vi "002_WarningLog.vi"(11 "Queue Ref":T1={"UI"=refnum, "Message"=refnum, "Data"=refnum, "Caller"=refnum, "Name"="000 Common", "Data Path"=path "", "Class Path"=path "", "SubPanel"=refnum, "Project Name"="", "MNT"="", "Title"="", "Data Source"=refnum, "Queue List"={}, "VI"=refnum, "UE"=refnum}) -> ()   [LabVIEW 2020]
uses:
  Alin/QMH/000 Module Data Type.ctl
  Alin/QMH/Queue Message.ctl
  9999 SubVI/Global/Data Global/Data Global Mode.ctl
  <vilib>/Utility/miscctls.llb/LVRowAndColumnUnsignedTypeDef.ctl
  9999 SubVI/Global/Data Global/SDQ Data Type.ctl
  <vilib>/Utility/file.llb/Read Delimited Spreadsheet (string).vi
panel:
  out "QN":i32
  out "Log Title":bool
  out "Warning Title":bool
  in  "Log Select":enum32{"History", "Real"}(radio)
  in  "Search Log":bool
  in  "Log Stop Time":timestamp caption="结束时间" format="%<%x %.0X>T"
  in  "Log Start Time":timestamp caption="开始时间" format="%<%x %.0X>T"
  in  "Warning Edit":bool
  in  "Warning Query":bool
  in  "Warning Stop Time":timestamp caption="结束时间" format="%<%x %X>T"
  in  "Warning Start Time":timestamp caption="开始时间" format="%<%x %.0X>T"
  in  "Warning Select":enum32{"History", "Real"}(radio)
  in  "Panel Show":bool
  in  "Operate":i32(listbox) caption="操作日志"
  in  "Warning":i32(listbox) caption="报警日志"
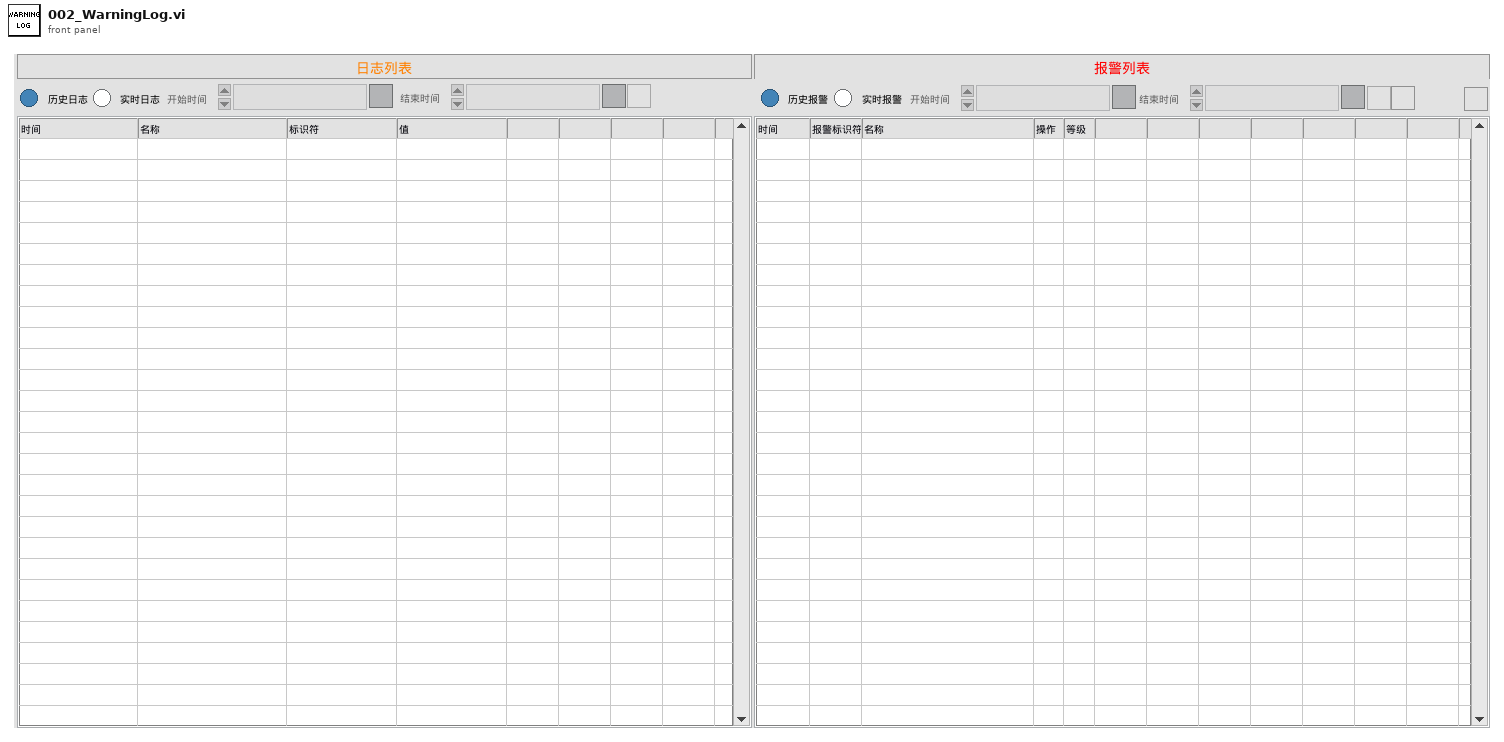
[diagram p1: front panel]
types:
  T1 = typedef "000 Module Data Type.ctl" = cluster{"UI":refnum<queue>, "Message":refnum<queue>, "Data":refnum<queue>, "Caller":refnum<queue>, "Name":string, "Data Path":path, "Class Path":path, "SubPanel":refnum<vi>, "Project Name":string, "MNT":string, "Title":string, "Data Source":refnum<queue>, "Queue List":map{string, refnum<queue>}, "VI":refnum<vi>, "UE":refnum<user-event>}
  T2 = typedef "SDQ Data Type.ctl" = cluster{"CAN Length":string, "CAN Name":string, "CAN ID":string, "CAN Type":string, "Test Item":string, "Byte Order":string, "Instruction":string, "Control Type":string, "Group":string, "Offset":dbl, "Coefficient":dbl, "Write Enable":bool, "Lable Type":string, "Key?":string, "Set Value":string, "Upper":dbl, "Lower":dbl, "Unit":string, "Formula":string, "Test Item Type":string, "Length":i32, "Address":string, "Name":string, "Identifier":string, "Data Type":string, "Enumerate?":string, "Enumerate List":string, "Data":string, "Source":string}
  T3 = cluster{"Queue Ref":T1, "Receive Data":map{string, T2}, "Log":string[][], "History Log":string[][], "Warning":string[][], "History Warning":string[][], "Delay":cluster{"Count Time(ms)":u32, "Delay Time(ms)":u32}, "Step":cluster{"Warning Judge":string, "Delay":string}}
  T4 = typedef "LVRowAndColumnUnsignedTypeDef.ctl" = cluster{"Row":u32, "Column":u32}
  T5 = enum8{"Enabled", "Disabled", "Disabled and Grayed Out"}
  T6 = typedef "eventvkey.ctl" = enum16{"ASCII", "Enter", "Return", "Shift", "Ctrl", "Alt", "Cmd", "Opt", "Caps", "NumLock", "Clear", "Break", "Up", "Down", "Left", "Right", "Insert", "Delete", "Home", "End", "PageUp", "PageDown", "Escape", "Help", "Pause", "ScrollLock", "F1", "F2", "F3", "F4", "F5", "F6", "F7", "F8", "F9", "F10", "F11", "F12", "F13", "F14", "F15", "F16", "F17", "F18", "F19", "F20", "F21", "F22", "F23", "F24", "Play", "VolumeUp", "VolumeDown", "Mute", "Two Byte Char"}
  T7 = cluster{"Shift":bool, "Ctrl":bool, "Alt":bool, "Cmd":bool, "Opt":bool}
  T8 = cluster{"Queue List":map{string, refnum<queue>}, "SubPanel":refnum<vi>, "Active Panel":string, "Queue Ref":T1, "Project Name":string}
  T9 = typedef "Data Global Mode.ctl" = enum16{"Init", "Read", "Write", "Write Data", "Load"}
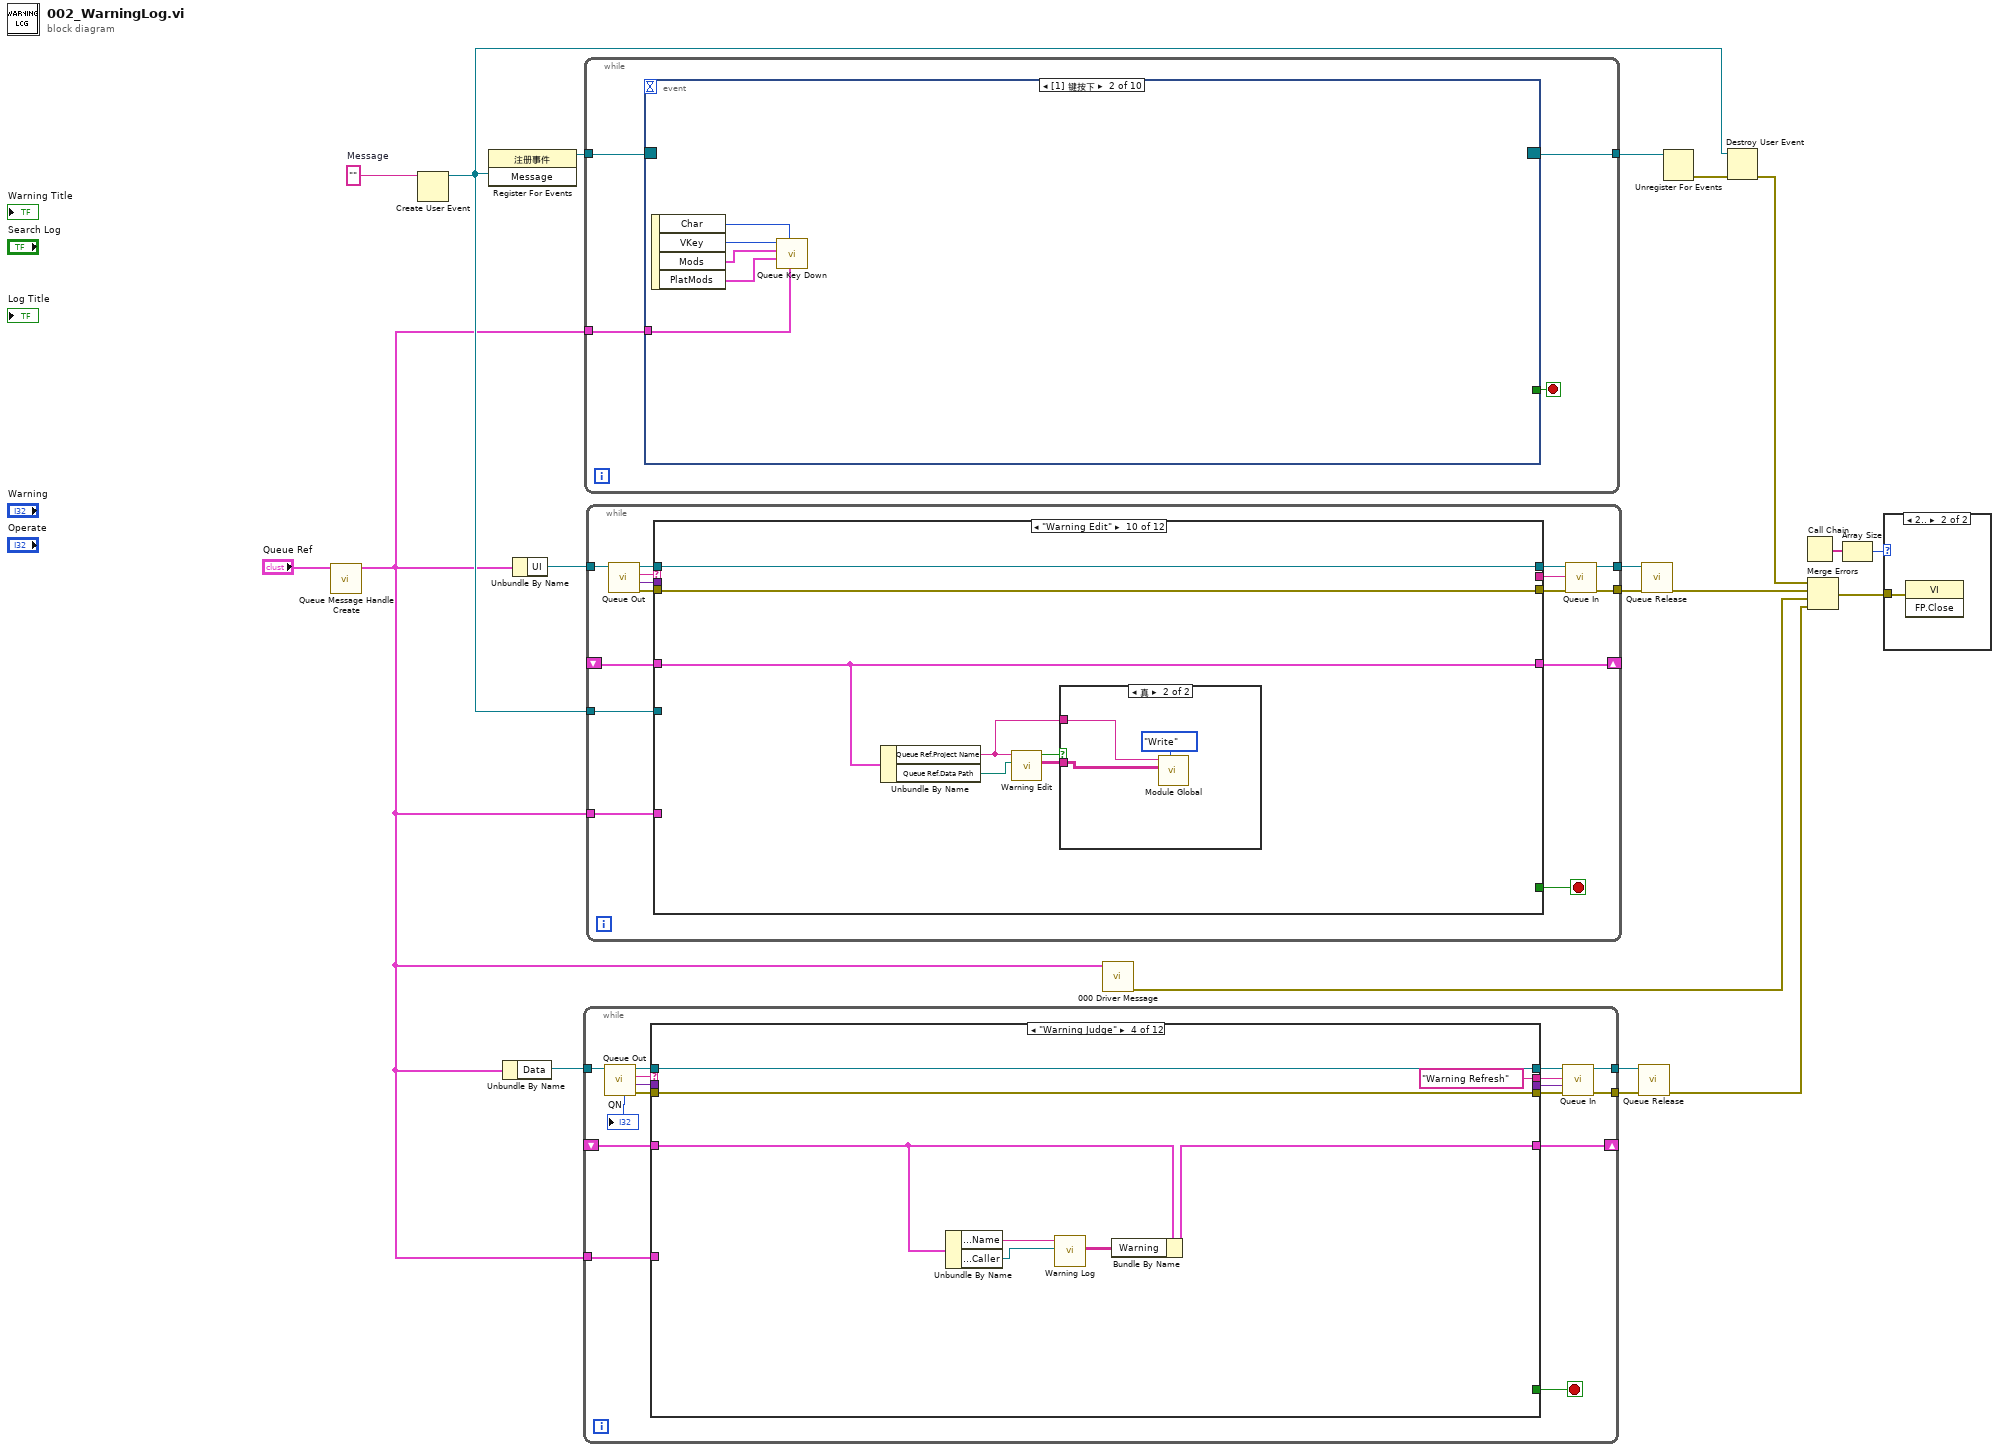
[diagram p0: block diagram]
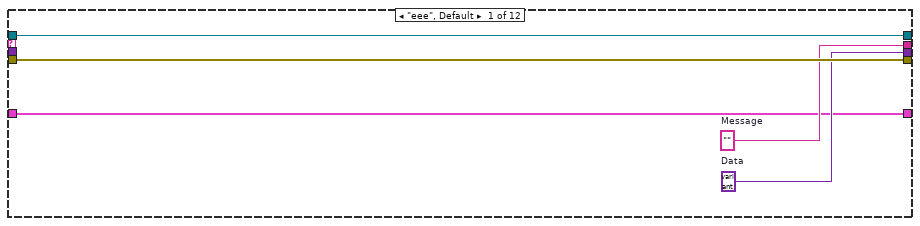
[diagram p2: hidden frame]
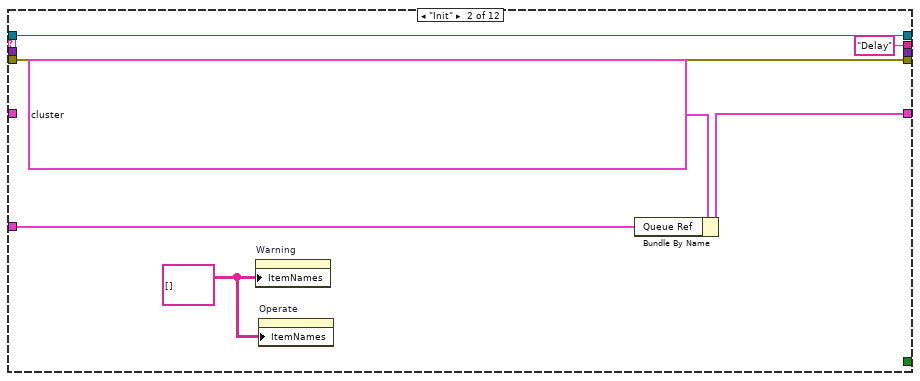
[diagram p3: hidden frame]
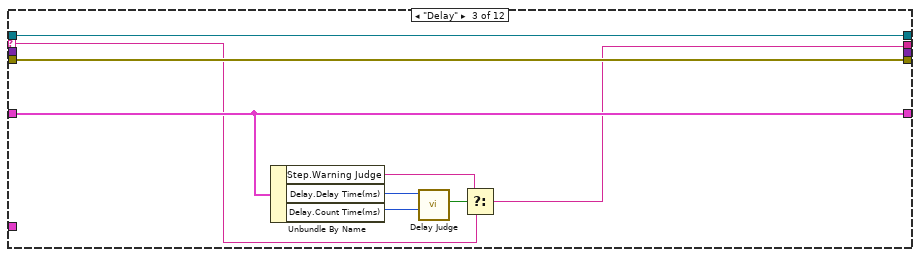
[diagram p4: hidden frame]
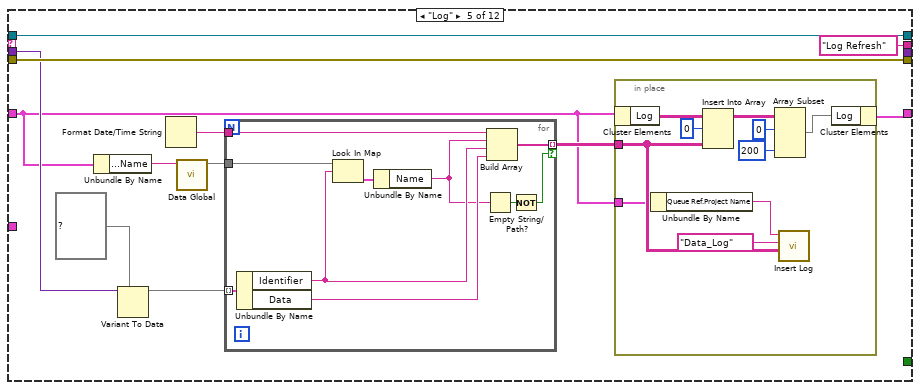
[diagram p5: hidden frame]
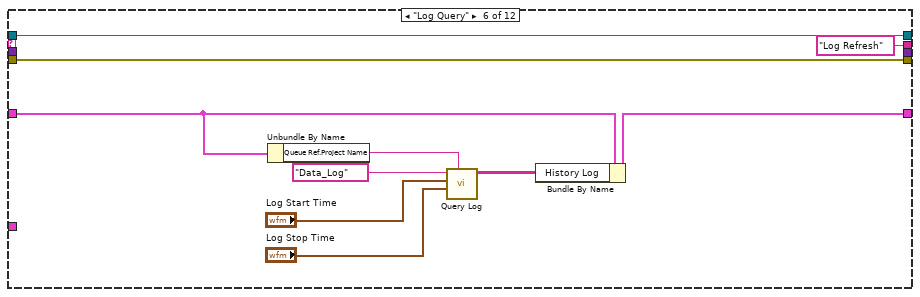
[diagram p6: hidden frame]
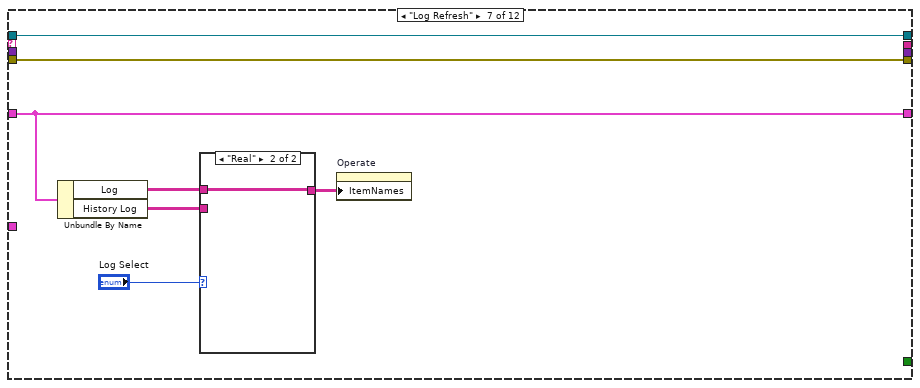
[diagram p7: hidden frame]
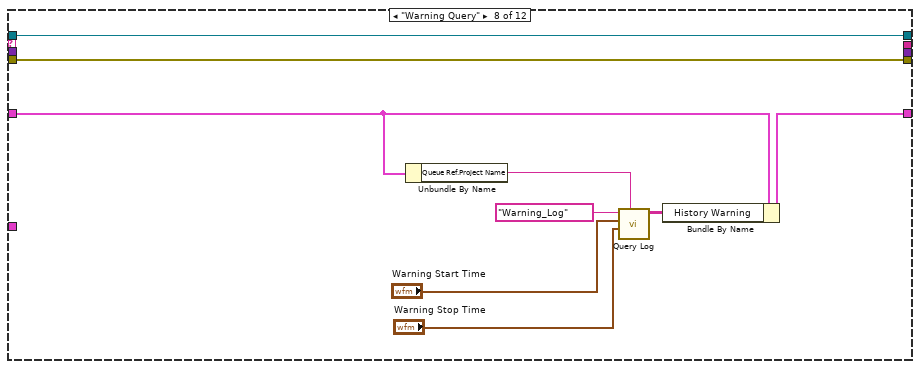
[diagram p9: hidden frame]
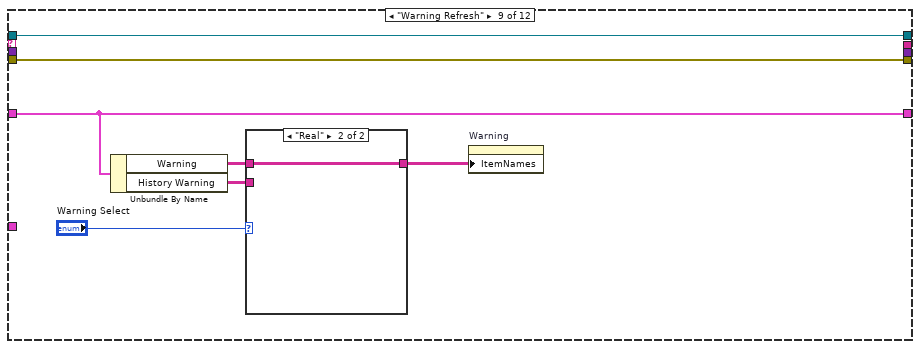
[diagram p10: hidden frame]
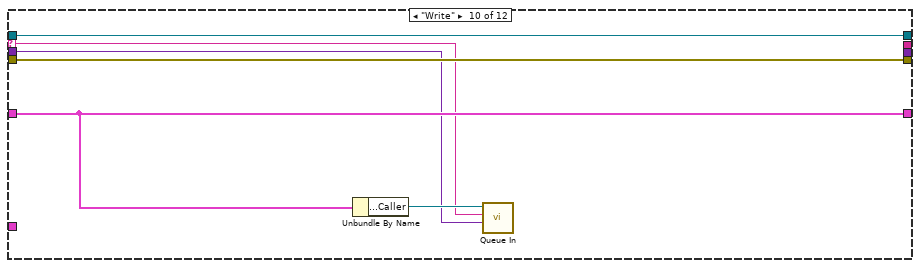
[diagram p12: hidden frame]
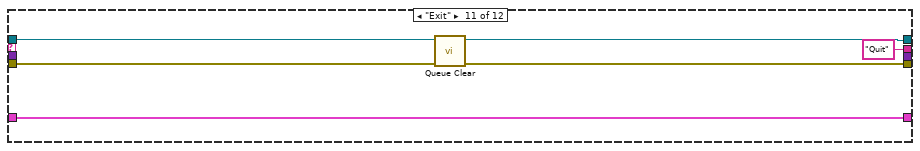
[diagram p13: hidden frame]
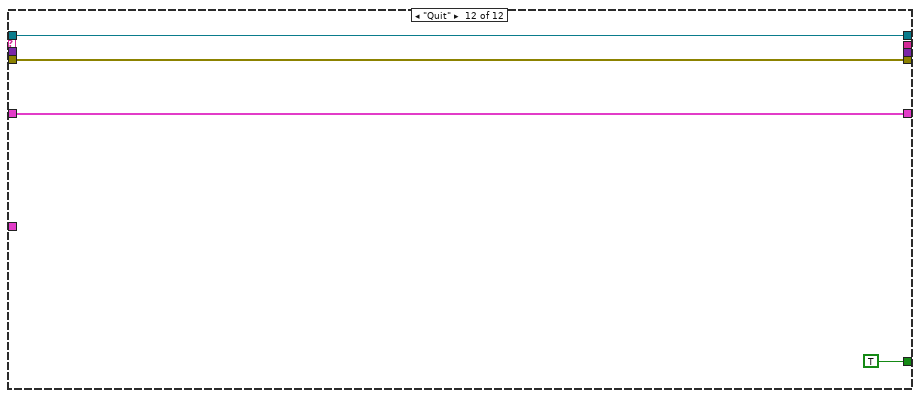
[diagram p14: hidden frame]
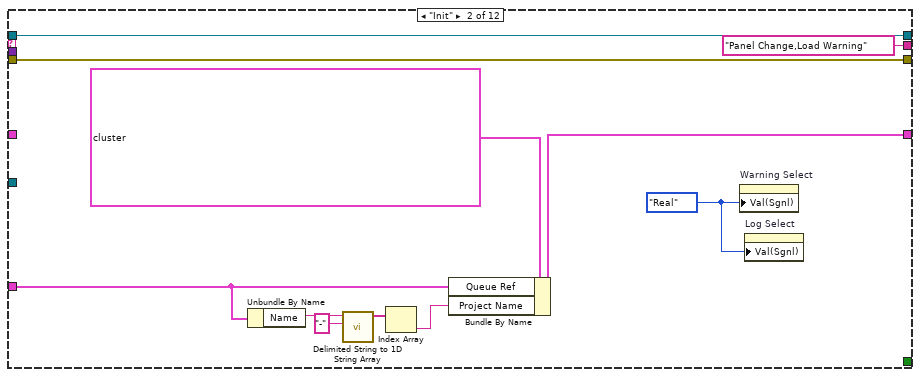
[diagram p17: hidden frame]
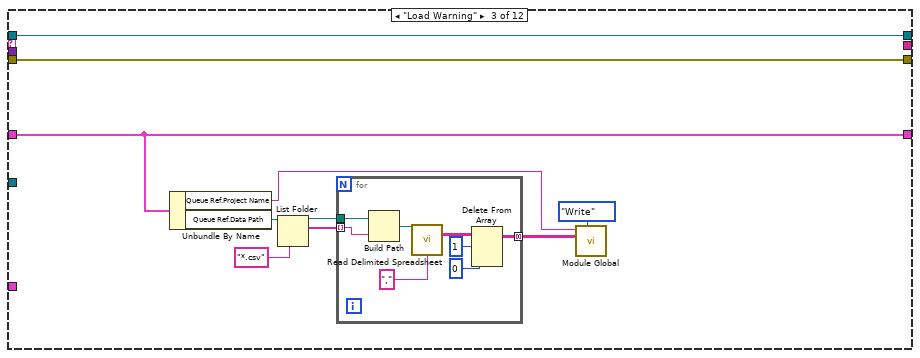
[diagram p18: hidden frame]
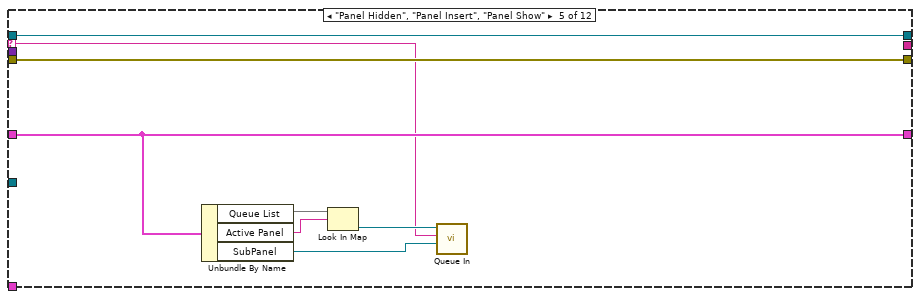
[diagram p20: hidden frame]
diagram:
  w3 = ""  # Message
  n1 = call "Queue Message Handle Create.vi"("Queue Ref In"="Queue Ref") -> ("Queue Ref Out"=w2:T1)  [unwired: 9 in, 1 out]
  n2 = Create User Event(user event datatype=w3) -> (user event=w7:refnum<user-event>)  [unwired: 1 in, 1 out]
  n3 = register-events(w7) -> (reference out=w4:refnum<event-registration>)  [unwired: 2 in, 1 out]
  n4 = Unbundle By Name(w2) -> ("Data"=w18:refnum<queue>)
  n5 = Unbundle By Name(w2) -> ("UI"=w10:refnum<queue>)
  n6 = while {
    tunnel: w18 -> [w32]
    tunnel: [w29] -> w16
    tunnel: [w28] -> w17
    shift-right: [w24] -> _
    shift-left: _ -> [w23]
    tunnel: w2 -> [w22]
    stop <- w36 stop-if-true
    n7 = call "Queue Out.vi"("Queue In"=w32) -> ("error out"=w35:errorcluster, "Data"=w33:variant, "Message"=w34:string, "Queue Out"=w31:refnum<queue>, "Queue NUmber"=→"QN":i32)  [unwired: 6 in]
    n8 = case shown="\"Warning Judge\"" w34 {
      selector: w34 -> [_ _ w51 _ _ _ _ _ _ w136 _ _]
      tunnel: w31 -> [w41 w48 w57 w65 w77 w107 w114 w125 w132 w140 w145 w149]
      tunnel: w35 -> [w40 w47 w56 w64 w76 w106 w113 w124 w131 w139 w143 w150]
      tunnel: [w41 w48 w57 w65 w77 w107 w114 w125 w132 w140 w144 w149] -> w30
      tunnel: [w40 w47 w56 w64 w76 w106 w113 w124 w131 w139 w142 w150] -> w27
      tunnel: [w39 "Delay" ("Message") w50 "Warning Refresh" ("Message") "Log Refresh" ("Message") "Log Refresh" ("Message") _ _ _ _ "Quit" _] -> w26
      tunnel: [_ _ _ _ _ _ _ _ _ _ _ TRUE] -> w36
      tunnel: [w38 _ _ _ _ _ _ _ _ _ _ _] -> w25
      tunnel: w33 -> [_ _ _ _ w75 _ _ _ _ w135 _ _]
      tunnel: [w37 w45 w54 w61 w69 w102 w112 w122 w129 w138 w141 w147] -> w24
      tunnel: w23 -> [w37 _ w54 w59 w66 w105 w112 w123 w129 w138 w141 w147]
      tunnel: w22 -> [_ w44 _ _ _ _ _ _ _ _ _ _]
      frame "eee", Default {
        w38 = variant  # Data
        w39 = ""  # Message
      }
      frame "Init" {
        w43 = string[][] [] ("项名")
        n9 = property on="Warning" class="MCListbox (严格)"("ItemNames"=w43) -> ()  [unwired: 2 in, 2 out]
        n10 = property on="Operate" class="MCListbox (严格)"("ItemNames"=w43) -> ()  [unwired: 2 in, 2 out]
        n11 = Bundle By Name(cluster=T3 {"Queue Ref"={"UI"=refnum, "Message"=refnum, "Data"=refnum, "Caller"=refnum, "Name"="", "Data Path"=path "", "Class Path"=path "", "SubPanel"=refnum, "Project Name"="", "MNT"="", "Title"="", "Data Source"=refnum, "Queue List"={}, "VI"=refnum, "UE"=refnum}, "Receive Data"={}, "Log"=[], "History Log"=[], "Warning"=[], "History Warning"=[], "Delay"={"Count Time(ms)"=500, "Delay Time(ms)"=250}, "Step"={"Warning Judge"="Warning Judge,Delay", "Delay"="Delay"}}, "Queue Ref"=w44) -> (w45:T3)
      }
      frame "Delay" {
        n12 = Unbundle By Name(w54) -> ("Step.Warning Judge"=w49:string, "Delay.Delay Time(ms)"=w53:u32, "Delay.Count Time(ms)"=w52:u32)
        n13 = call "Delay Judge.vi"("Delay Time(ms)"=w52, "Count Time(ms)"=w53) -> ("Time Out?"=w55:bool)  [unwired: 5 in, 4 out]
        n14 = Select(t=w49, s=w55, f=w51) -> (s? t:f=w50:string)
      }
      frame "Warning Judge" {
        n15 = Unbundle By Name(w59) -> ("Queue Ref.Name"=w63:string, "Queue Ref.Caller"=w58:refnum<queue>)
        n16 = call "Warning Log.vi"("Caller"=w58, "Name"=w63) -> ("Current"=w60:string[][])  [unwired: 9 in]
        n17 = Bundle By Name(cluster=w59, "Warning"=w60) -> (w61:T3)
      }
      frame "Log" {
        n18 = Unbundle By Name(w66) -> ("Queue Ref.Name"=w72:string)
        n19 = Variant To Data(type=map{string, string} {} ("数据"), Variant=w75) -> (data=w73:map{string, string})  [unwired: 1 in, 1 out]
        n20 = Format Date/Time String() -> (date/time string=w70:string)  [unwired: 3 in]
        n21 = call "Data Global.vi"("Name"=w72) -> ("Data Out"=w71:map{string, T2})  [unwired: 7 in, 3 out]
        n22 = for {
          tunnel: w73 -> [w97] mode=indexing
          tunnel: w71 -> [w96]
          tunnel: w70 -> [w94]
          tunnel: [w91] -> w68 mode=indexing if=w88
          n23 = Unbundle By Name(w97) -> ("Identifier"=w93:string, "Data"=w92:string)
          n24 = Look In Map(map=w96, key=w93) -> (value=w95:T2)  [unwired: 1 in, 1 out]
          n25 = Unbundle By Name(w95) -> ("Name"=w90:string)
          n26 = Empty String/Path?(string/path=w90) -> (empty?=w89:bool)
          n27 = Build Array(w94, w90, w93, w92) -> (w91:string[])
          n28 = Not(x=w89) -> (.not. x?=w88:bool)
        }
        n29 = in-place {
          in-place-border: w68 -> [w81]
          in-place-border: w66 -> [w80]
          n30 = in-place-cluster #1(w66) -> ("Log"=w87:string[][])
          n31 = Unbundle By Name(w80) -> ("Queue Ref.Project Name"=w79:string)
          n32 = Insert Into Array(array=w87, index (row)=0 ("索引 (行)"), new element=w81) -> (w85:string[][])  [unwired: 1 in]
          n33 = Array Subset(array=w85, index (row)=0 ("索引"), length (row)=200 ("长度")) -> (w82:string[][])  [unwired: 2 in]
          n34 = call "Insert Log.vi"("Data"=w81, "Table"="Data_Log", "Project"=w79) -> ()  [unwired: 8 in, 1 out]
          n35 = in-place-cluster #1("Log"=w82) -> (w69:T3)
        }
      }
      frame "Log Query" {
        n36 = Unbundle By Name(w105) -> ("Queue Ref.Project Name"=w99:string)
        n37 = call "Query Log.vi"("Project"=w99, "Stop Time"="Log Stop Time", "Start Time"="Log Start Time", "Table"="Data_Log") -> ("data"=w101:string[][])  [unwired: 6 in, 1 out]
        n38 = Bundle By Name(cluster=w105, "History Log"=w101) -> (w102:T3)
      }
      frame "Log Refresh" {
        n39 = Unbundle By Name(w112) -> ("Log"=w110:string[][], "History Log"=w109:string[][])
        n40 = case shown="\"Real\"" "Log Select" {
          tunnel: w110 -> [_ w116]
          tunnel: w109 -> [w115 _]
          tunnel: [w115 w116] -> w108
          frame "History", Default {
          }
          frame "Real" {
          }
        }
        n41 = property on="Operate" class="MCListbox (严格)"("ItemNames"=w108) -> ()  [unwired: 2 in, 2 out]
      }
      frame "Warning Query" {
        n42 = Unbundle By Name(w123) -> ("Queue Ref.Project Name"=w120:string)
        n43 = call "Query Log.vi"("Project"=w120, "Stop Time"="Warning Stop Time", "Start Time"="Warning Start Time", "Table"="Warning_Log") -> ("data"=w121:string[][])  [unwired: 6 in, 1 out]
        n44 = Bundle By Name(cluster=w123, "History Warning"=w121) -> (w122:T3)
      }
      frame "Warning Refresh" {
        n45 = Unbundle By Name(w129) -> ("Warning"=w128:string[][], "History Warning"=w127:string[][])
        n46 = case shown="\"Real\"" "Warning Select" {
          tunnel: w128 -> [_ w134]
          tunnel: w127 -> [w133 _]
          tunnel: [w133 w134] -> w126
          frame "History", Default {
          }
          frame "Real" {
          }
        }
        n47 = property on="Warning" class="MCListbox (严格)"("ItemNames"=w126) -> ()  [unwired: 2 in, 2 out]
      }
      frame "Write" {
        n48 = Unbundle By Name(w138) -> ("Queue Ref.Caller"=w137:refnum<queue>)
        n49 = call "Queue In.vi"("Data"=w135, "Message"=w136, "Queue In"=w137) -> ()  [unwired: 7 in, 2 out]
      }
      frame "Exit" {
        n50 = call "Queue Clear.vi"("error in (no error)"=w143, "Queue In"=w145) -> ("error out"=w142:errorcluster, "Queue Out"=w144:refnum<queue>)  [unwired: 8 in]
      }
      frame "Quit" {
      }
    }
    n51 = call "Queue In.vi"("error in (no error)"=w27, "Data"=w25, "Message"=w26, "Queue In"=w30) -> ("error out"=w28:errorcluster, "Queue Out"=w29:refnum<queue>)  [unwired: 6 in]
  }
  n52 = while {
    tunnel: w4 -> [w154]
    tunnel: [w152] -> w5
    tunnel: w2 -> [w151]
    stop <- w153 stop-if-true
    n53 = event shown="[1] 键按下" {
      selector: w154 -> [_ _ _ _ _ _ _ _ _ _]
      dyn-events: [_ _ _ _ _ _ _ _ _ _] -> w152
      timeout: _ -> [_ _ _ _ _ _ _ _ _ _]
      tunnel: [_ _ _ w163 _ _ _ _ _ _] -> w153
      tunnel: w151 -> [_ w157 w162 _ w167 w175 w199 w219 w223 w226]
      event Timeout {
        n54 = event-data() -> ()  [unwired: 1 in, 1 out]
      }
      event Key Down {
        n55 = event-data() -> ("Char"=w159:i16, "VKey"=w158:T6, "Mods"=w156:cluster{"Num Pad":bool, "Menu Key":bool}, "PlatMods"=w155:T7)  [unwired: 1 in]
        n56 = call "Queue Key Down.vi"("Queue Ref Out"=w157, "C"=w159, "Platform Key"=w155, "Group Key"=w156, "V Key"=w158) -> ()  [unwired: 6 in, 1 out]
      }
      event Panel Resize {
        n57 = event-data() -> ()  [unwired: 1 in, 1 out]
        n58 = Unbundle By Name(w162) -> ("Message"=w161:refnum<queue>)
        n59 = call "Queue In.vi"("Message"="Panel Change", "Queue In"=w161) -> ()  [unwired: 8 in, 2 out]
      }
      event User Event {
        n60 = event-data() -> ("Message"=w165:string)  [unwired: 1 in]
        n61 = Equal?(x=w165, y="Exit") -> (x = y?=w163:bool)
      }
      event Panel Close? {
        n62 = event-data() -> ()  [unwired: 1 in, 1 out]
        n63 = Unbundle By Name(w167) -> ("Message"=w166:refnum<queue>)
        n64 = Call Chain() -> (call chain=w170:string[])
        n65 = Array Size(array=w170) -> (size(s)=w169:i32)
        n66 = case shown="0, 默认" w169 {
          tunnel: ["Exit Prepare" ("Message") "Panel Hidden" ("Message")] -> w168
          frame 0, Default {
          }
          frame 2.. {
          }
        }
        n67 = call "Queue In.vi"("Message"=w168, "Queue In"=w166) -> ()  [unwired: 8 in, 2 out]
        n68 = event-data("Discard?"=TRUE ("放弃？")) -> ()  [unwired: 1 in, 1 out]
      }
      event "Warning Select": Value Change {
        n69 = event-data() -> ("NewVal"=w176:enum32{"History", "Real"})  [unwired: 1 in]
        n70 = case shown="\"Real\"" w176 {
          tunnel: [T5."Enabled" ("禁用") T5."Disabled and Grayed Out" ("禁用")] -> w177
          tunnel: w175 -> [w186 w190]
          frame "History", Default {
            n71 = Unbundle By Name(w186) -> ("Data"=w185:refnum<queue>)
            n72 = call "Queue In.vi"("Message"="Warning Query", "Queue In"=w185) -> ()  [unwired: 8 in, 2 out]
          }
          frame "Real" {
            n73 = Unbundle By Name(w190) -> ("Data"=w189:refnum<queue>)
            n74 = Get Date/Time In Seconds() -> (seconds since 1Jan1904=w193:timestamp)
            n75 = Subtract(x=w193, y=3600.0) -> (x-y=w192:timestamp)
            n76 = call "Queue In.vi"("Message"="Warning Refresh", "Queue In"=w189) -> ()  [unwired: 8 in, 2 out]
            n77 = local write "Warning Start Time"(w192) -> ()
            n78 = local write "Warning Stop Time"(w193) -> ()
          }
        }
        n79 = property on="Warning" class="MCListbox (严格)"("TopLeft"=T4 {"Row"=0, "Column"=0} ("左上可见单元格")) -> ()  [unwired: 2 in, 2 out]
        n80 = control-ref of="Warning Stop Time"() -> (w180:refnum<vi>)
        n81 = control-ref of="Warning Start Time"() -> (w179:refnum<vi>)
        n82 = control-ref of="Warning Query"() -> (w181:refnum<vi>)
        n83 = Build Array(w181, w180, w179) -> (w178:refnum<vi>[])
        n84 = for {
          tunnel: w178 -> [w183] mode=indexing
          tunnel: w177 -> [w182]
          n85 = property class="Ctl"(reference=w183, "DisabledEnum"=w182) -> ()  [unwired: 1 in, 2 out]
        }
      }
      event "Log Select": Value Change {
        n86 = event-data() -> ("NewVal"=w200:enum32{"History", "Real"})  [unwired: 1 in]
        n87 = case shown="\"Real\"" w200 {
          tunnel: [T5."Enabled" ("禁用") T5."Disabled and Grayed Out" ("禁用")] -> w201
          tunnel: w199 -> [w210 w214]
          frame "History", Default {
            n88 = Get Date/Time In Seconds() -> (seconds since 1Jan1904=w206:timestamp)
            n89 = Unbundle By Name(w210) -> ("Data"=w209:refnum<queue>)
            n90 = call "Queue In.vi"("Message"="Log Query", "Queue In"=w209) -> ()  [unwired: 8 in, 2 out]
            n91 = Subtract(x=w206, y=3600.0) -> (x-y=w207:timestamp)
            n92 = local write "Log Start Time"(w207) -> ()
            n93 = local write "Log Stop Time"(w206) -> ()
          }
          frame "Real" {
            n94 = Unbundle By Name(w214) -> ("Data"=w213:refnum<queue>)
            n95 = call "Queue In.vi"("Message"="Log Refresh", "Queue In"=w213) -> ()  [unwired: 8 in, 2 out]
          }
        }
        n96 = control-ref of="Search Log"() -> (w197:refnum<vi>)
        n97 = control-ref of="Log Stop Time"() -> (w198:refnum<vi>)
        n98 = control-ref of="Log Start Time"() -> (w196:refnum<vi>)
        n99 = property on="Operate" class="MCListbox (严格)"("TopLeft"=T4 {"Row"=0, "Column"=0} ("左上可见单元格")) -> ()  [unwired: 2 in, 2 out]
        n100 = Build Array(w197, w198, w196) -> (w202:refnum<vi>[])
        n101 = for {
          tunnel: w202 -> [w204] mode=indexing
          tunnel: w201 -> [w203]
          n102 = property class="Ctl"(reference=w204, "DisabledEnum"=w203) -> ()  [unwired: 1 in, 2 out]
        }
      }
      event "Warning Edit": Value Change {
        n103 = event-data() -> ("CtlRef"=w218:refnum<vi>)  [unwired: 1 in]
        n104 = property class="Bool"(reference=w218) -> ("Label.Text"=w216:string)  [unwired: 1 in, 2 out]
        n105 = Unbundle By Name(w219) -> ("UI"=w217:refnum<queue>)
        n106 = call "Queue In.vi"("Message"=w216, "Queue In"=w217) -> ()  [unwired: 8 in, 2 out]
      }
      event "Panel Show": Value Change {
        n107 = event-data() -> ("CtlRef"=w221:refnum<vi>)  [unwired: 1 in]
        n108 = Unbundle By Name(w223) -> ("Message"=w222:refnum<queue>)
        n109 = property class="Bool"(reference=w221) -> ("Label.Text"=w220:string)  [unwired: 1 in, 2 out]
        n110 = call "Queue In.vi"("Message"=w220, "Queue In"=w222) -> ()  [unwired: 8 in, 2 out]
      }
      event "Warning Query": Value Change {
        n111 = event-data() -> ("CtlRef"=w227:refnum<vi>)  [unwired: 1 in]
        n112 = Unbundle By Name(w226) -> ("Data"=w225:refnum<queue>)
        n113 = property class="Bool"(reference=w227) -> ("Label.Text"=w224:string)  [unwired: 1 in, 2 out]
        n114 = call "Queue In.vi"("Message"=w224, "Queue In"=w225) -> ()  [unwired: 8 in, 2 out]
      }
    }
  }
  n115 = while {
    tunnel: w10 -> [w237]
    tunnel: [w234] -> w8
    tunnel: [w233] -> w9
    tunnel: w7 -> [w241]
    tunnel: w2 -> [w230]
    shift-right: [w229] -> _
    shift-left: _ -> [w228]
    stop <- w242 stop-if-true
    n116 = call "Queue Out.vi"("Queue In"=w237) -> ("error out"=w240:errorcluster, "Data"=w238:variant, "Message"=w239:string, "Queue Out"=w236:refnum<queue>)  [unwired: 6 in, 1 out]
    n117 = case shown="\"Warning Edit\"" w239 {
      selector: w239 -> [_ _ _ _ w280 _ _ w299 _ _ w318 _]
      tunnel: w236 -> [w245 w256 w266 w277 w285 w288 w293 w303 w306 w313 w326 w334]
      tunnel: w240 -> [w244 w255 w265 w276 w284 w287 w292 w302 w305 w312 w324 w335]
      tunnel: [w245 w256 w266 w277 w285 w288 w293 w303 w306 w313 w325 w334] -> w235
      tunnel: [w244 w255 w265 w276 w284 w287 w292 w302 w305 w312 w323 w335] -> w232
      tunnel: [_ "Panel Change,Load Warning" _ _ _ _ _ _ _ _ "Quit" _] -> w231
      tunnel: [_ _ _ _ _ _ _ _ _ _ _ TRUE] -> w242
      tunnel: w241 -> [_ _ _ _ _ _ _ _ _ _ w328 _]
      tunnel: w238 -> [_ _ _ _ _ _ w289 _ _ _ _ _]
      tunnel: w230 -> [_ w252 _ _ _ _ _ w301 _ _ w322 _]
      tunnel: [w243 w253 w260 w275 w283 w286 w290 w298 w304 w311 w317 w332] -> w229
      tunnel: w228 -> [w243 _ w260 w275 w283 w286 w291 w298 w304 w311 w317 w332]
      frame "eee", Default {
      }
      frame "Init" {
        w247 = enum32{"History", "Real"}."Real" ("Warning Select")
        n118 = Unbundle By Name(w252) -> ("Name"=w251:string)
        n119 = call <vilib>:"Delimited String to 1D String Array.vi"("delimiter"="-", "delimited string"=w251) -> ("string array"=w249:string[])  [unwired: 9 in]
        n120 = Index Array(array=w249) -> (element=w248:string)  [unwired: 1 in]
        n121 = Bundle By Name(cluster=T8 {"Queue List"={}, "SubPanel"=refnum, "Active Panel"="", "Queue Ref"={"UI"=refnum, "Message"=refnum, "Data"=refnum, "Caller"=refnum, "Name"="", "Data Path"=path "", "Class Path"=path "", "SubPanel"=refnum, "Project Name"="", "MNT"="", "Title"="", "Data Source"=refnum, "Queue List"={}, "VI"=refnum, "UE"=refnum}, "Project Name"=""}, "Queue Ref"=w252, "Project Name"=w248) -> (w253:T8)
        n122 = property on="Warning Select" class="RadioBtnsControl (严格)"("Val(Sgnl)"=w247) -> ()  [unwired: 2 in, 2 out]
        n123 = property on="Log Select" class="RadioBtnsControl (严格)"("Val(Sgnl)"=w247) -> ()  [unwired: 2 in, 2 out]
      }
      frame "Load Warning" {
        n124 = Unbundle By Name(w260) -> ("Queue Ref.Project Name"=w257:string, "Queue Ref.Data Path"=w264:path)
        n125 = List Folder(path=w264, pattern="*.csv" ("类型")) -> (path out=w262:path, filenames=w263:string[])  [unwired: 2 in, 2 out]
        n126 = for {
          tunnel: w263 -> [w273] mode=indexing
          tunnel: w262 -> [w274]
          tunnel: [w267] -> w258 mode=concatenating
          n127 = Build Path(base path=w274, name or relative path=w273) -> (appended path=w272:path)
          n128 = call-poly <vilib>:"Read Delimited Spreadsheet.vi"("file path (dialog if empty)"=w272, "delimiter (\\t)"="," ("delimiter (\\t)")) -> ("all rows"=w270:string[][])  [unwired: 8 in, 5 out]
          n129 = Delete From Array(array=w270, length=1 ("长度"), index (row)=0 ("索引 (行)")) -> (array with subset deleted=w267:string[][])  [unwired: 1 in, 1 out]
        }
        n130 = call "Module Global.vi"("Operate"=Data_Global_Mode."Write", "Warning List"=w258, "Project"=w257) -> ()  [unwired: 7 in, 2 out]
      }
      frame "====System====" {
      }
      frame "Panel Hidden", "Panel Insert", "Panel Show" {
        n131 = Unbundle By Name(w283) -> ("Queue List"=w282:map{string, refnum<queue>}, "Active Panel"=w279:string, "SubPanel"=w278:refnum<vi>)
        n132 = Look In Map(map=w282, key=w279) -> (value=w281:refnum<queue>)  [unwired: 1 in, 1 out]
        n133 = call "Queue In.vi"("Data"=w278, "Message"=w280, "Queue In"=w281) -> ()  [unwired: 7 in, 2 out]
      }
      frame "Panel Change" {
        n134 = call "MCList Adjust.vi"() -> ()  [unwired: 11 in, 1 out]
      }
      frame "Send Client Refer" {
        n135 = in-place {
          in-place-border: w289 -> [w295]
          n136 = in-place-cluster #2(w291) -> ("Queue List"=w294:map{string, refnum<queue>})
          n137 = Variant To Data(type=w294, Variant=w295) -> (data=w296:map{string, refnum<queue>})  [unwired: 1 in, 1 out]
          n138 = in-place-cluster #2("Queue List"=w296) -> (w290:T8)
        }
      }
      frame "Client Delete", "Client Launch" {
        n139 = Unbundle By Name(w301) -> ("Message"=w300:refnum<queue>)
        n140 = Unbundle By Name(w298) -> ("Active Panel"=w297:string)
        n141 = call "Queue In.vi"("Data"=w297, "Message"=w299, "Queue In"=w300) -> ()  [unwired: 7 in, 2 out]
      }
      frame "====User====" {
      }
      frame "Warning Edit" {
        n142 = Unbundle By Name(w311) -> ("Queue Ref.Project Name"=w309:string, "Queue Ref.Data Path"=w308:path)
        n143 = call "Warning Edit.vi"("Data Path"=w308, "Project"=w309) -> ("Warning Data"=w307:string[][], "OK?"=w310:bool)  [unwired: 8 in]
        n144 = case shown="真" w310 {
          tunnel: w309 -> [_ w315]
          tunnel: w307 -> [_ w314]
          frame False {
          }
          frame True {
            n145 = call "Module Global.vi"("Operate"=Data_Global_Mode."Write", "Warning List"=w314, "Project"=w315) -> ()  [unwired: 7 in, 2 out]
          }
        }
      }
      frame "Exit" {
        n146 = Unbundle By Name(w322) -> ("Message"=w321:refnum<queue>, "Data"=w320:refnum<queue>)
        n147 = Build Array(w321, w320) -> (w319:refnum<queue>[])
        n148 = for {
          tunnel: w319 -> [w331] mode=indexing
          tunnel: w318 -> [w330]
          n149 = call "Queue In.vi"("First"=TRUE, "Message"=w330, "Queue In"=w331) -> ()  [unwired: 7 in, 2 out]
        }
        n150 = Generate User Event(user event=w328, event data cluster=w318) -> ()  [unwired: 2 in, 2 out]
        n151 = call "Queue Clear.vi"("error in (no error)"=w324, "Queue In"=w326) -> ("error out"=w323:errorcluster, "Queue Out"=w325:refnum<queue>)  [unwired: 8 in]
      }
      frame "Quit" {
      }
    }
    n152 = call "Queue In.vi"("error in (no error)"=w232, "Message"=w231, "Queue In"=w235) -> ("error out"=w233:errorcluster, "Queue Out"=w234:refnum<queue>)  [unwired: 7 in]
  }
  n153 = call "000 Driver Message.vi"("Queue In"=w2) -> ("error out"=w19:errorcluster)  [unwired: 8 in, 2 out]
  n154 = call "Queue Release.vi"("error in (no error)"=w17, "Queue In"=w16) -> ("error out"=w20:errorcluster)  [unwired: 9 in]
  n155 = call "Queue Release.vi"("error in (no error)"=w9, "Queue In"=w8) -> ("error out"=w12:errorcluster)  [unwired: 9 in]
  n156 = Unregister For Events(event registration refnum=w5) -> (error out=w6:errorcluster)  [unwired: 1 in]
  n157 = Destroy User Event(user event=w7, error in=w6) -> (error out=w11:errorcluster)
  n158 = Call Chain() -> (call chain=w14:string[])
  n159 = Merge Errors(w11, w12, w19, w20) -> (w13:errorcluster)
  n160 = Array Size(array=w14) -> (size(s)=w15:i32)
  n161 = case shown="2.." w15 {
    tunnel: w13 -> [_ w336]
    frame 0, Default {
    }
    frame 2.. {
      n162 = invoke class="VI" method="FP.Close"(error in=w336) -> ()  [unwired: 2 in, 3 out]
    }
  }
